vi "RectangleToCenter.vi"(11 "input cluster":T1 {"Rotation" format="%.2f"; "Left" scale=0.0..1024.0; "Right" scale=0.0..1024.0}) -> (2 "y":dbl, 3 "x":dbl)   [LabVIEW 2011]
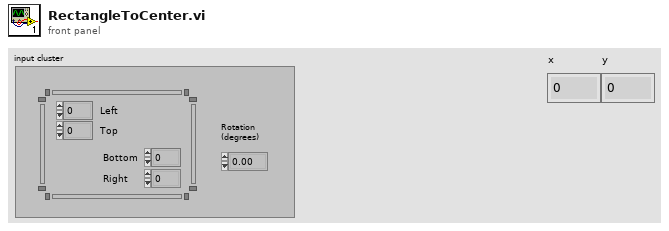
[diagram p1: front panel]
types:
  T1 = typedef "IMAQ Rectangle" = cluster{"Left":i32, "Top":i32, "Right":i32, "Bottom":i32, "Rotation":dbl}
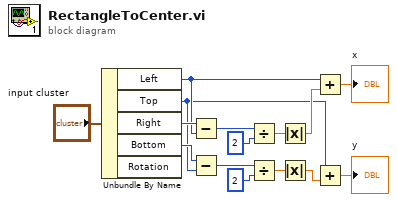
[diagram p0: block diagram]
diagram:
  n1 = Unbundle By Name("input cluster") -> ("Left"=w3:i32, "Top"=w1:i32, "Right"=w14:i32, "Bottom"=w11:i32)  [unwired: 1 out]
  n2 = Subtract(x=w14, y=w3) -> (x-y=w13:i32)
  n3 = Subtract(x=w11, y=w1) -> (x-y=w9:i32)
  n4 = Divide(x=w13, y=2) -> (x/y=w5:dbl)
  n5 = Divide(x=w9, y=2) -> (x/y=w6:dbl)
  n6 = Absolute Value(x=w5) -> (abs(x)=w4:dbl)
  n7 = Absolute Value(x=w6) -> (abs(x)=w2:dbl)
  n8 = Add(x=w3, y=w4) -> (x+y=→"x":dbl)
  n9 = Add(x=w1, y=w2) -> (x+y=→"y":dbl)
